vi "ClsGetStreamFailCounter.vi"(8 "error in (no error)":errorcluster, 11 "Connection In":u32) -> (0 "error out":errorcluster, 2 "number of failures":i32, 3 "Connection Out":u32)   [LabVIEW 2015]
doc: "Get Stream Fail Counter\n\nUnder normal operation, subVIs internally stays in sync with the device. However sometimes because of any reason, subVIs could be out of sync with device data stream (happens seldom). SubVIs then needs to resync with the device, this will cause data lost. If any data lost is detected at the client side, client could have a check with this function to see whether there is any problem between subVIs and the device.\n\nConnection In[Input]: the connection handle which is initially created by Open Connection subVI.\n\nNumber of Failures[Output]: Stream problem counter.\n\nConnection Out[Output]: the connection handle output which could be used for next subVI refering to the same connection."
uses:
  dependent dlls/CHRocodileDLL.dll
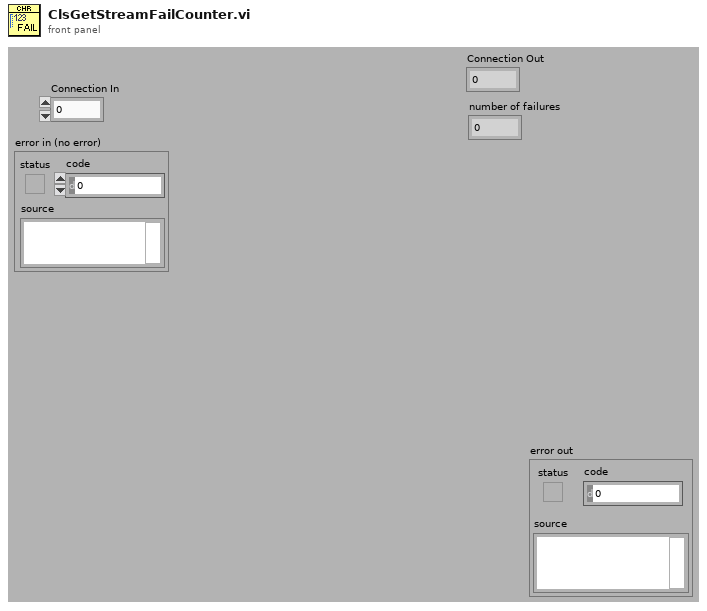
[diagram p1: front panel]
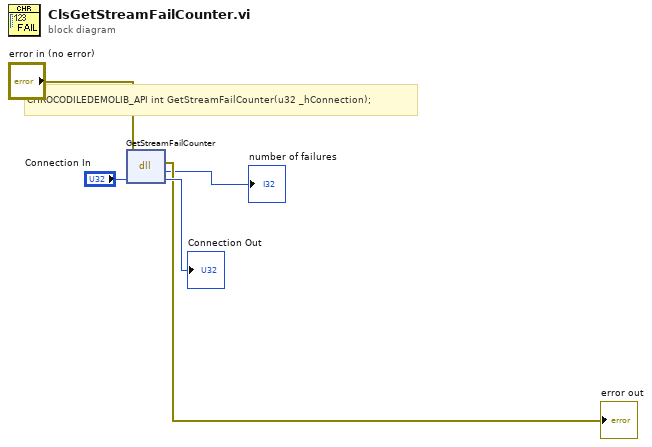
[diagram p0: block diagram]
diagram:
  # "CHROCODILEDEMOLIB_API int GetStreamFailCounter(u32 _hConnection);"
  n1 = dll-call lib="C:/Users/privat/Documents/ADP-SLA/Drop Impact Teststand/dependent dlls/CHRocodileDLL.dll" fn="GetStreamFailCounter"(error in="error in (no error)", "_hConnection"="Connection In") -> (error out=→"error out":errorcluster, "return type"=→"number of failures":i32, "_hConnection"=→"Connection Out":u32)  [unwired: 2 in, 1 out]
